vi "Main.vi"() -> ()   [LabVIEW 2016]
uses:
  Typedef/INS Data.ctl
  <vilib>/FPGAPlugInAG/roboRIO/niLvFpga_Open_roboRIO.vi
  <vilib>/rvi/interface/common/dynamic/niFpgaDynamicAddResources.vi
  <vilib>/FPGAPlugInAG/Dynamic/niLvFpga_Reset_Dynamic.vi
  <vilib>/Utility/error.llb/Error Cluster From Error Code.vi
  <vilib>/rvi/errors/niLvFpgaAdjustHostInterfaceError.vi
  <vilib>/myRIO/Common/Instrument Driver Framework/Utilities/vis/FPGA Ref Manager.vi
  <vilib>/myRIO/Common/Instrument Driver Framework/Utilities/vis/Ref Counter.vi
  <vilib>/FPGAPlugInAG/Dynamic/niLvFpga_Run_Dynamic.vi
  Shared resoruces/gear.vi
  Shared resoruces/Front Panel Control Variables.vi
  <vilib>/rvi/interface/nirviOpenFPGA/nirviOpenFPGA.xnode
  FPGA Bitfiles/AutoBikeMainFPGAbitfile.lvbitx
  <vilib>/rvi/interface/nirviMethod/nirviMethod.xnode
  <vilib>/rvi/interface/nirviReadWriteControl/nirviReadWriteControl.xnode
  <vilib>/rvi/interface/Simulation/niFpgaSimulationCallBeginRW.vi
  NiFpgaLv.dll
  <vilib>/myRIO/Instrument Drivers/Utilities/Utilities.lvlib
  Shared resoruces/Shared resources RT.lvlib
panel:
  in  "Reset Errors":bool
  in  "Send vel":bool
  in  "VEL":u16=850
  in  "UseGPS":bool=TRUE
  in  "Gear":enum16{"7", "6", "5", "4", "3", "2", "1"}(ring)=enum."3"
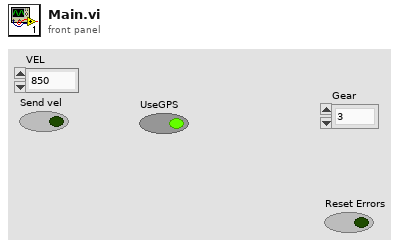
[diagram p1: front panel]
types:
  T1 = typedef "INS Data.ctl" = cluster{"Yaw":sgl, "Pitch":sgl, "Roll":sgl, "Lat":dbl, "Long":dbl, "Alt":dbl, "North":dbl, "East":dbl, "Down":dbl, "PosU":dbl, "VelU":dbl}
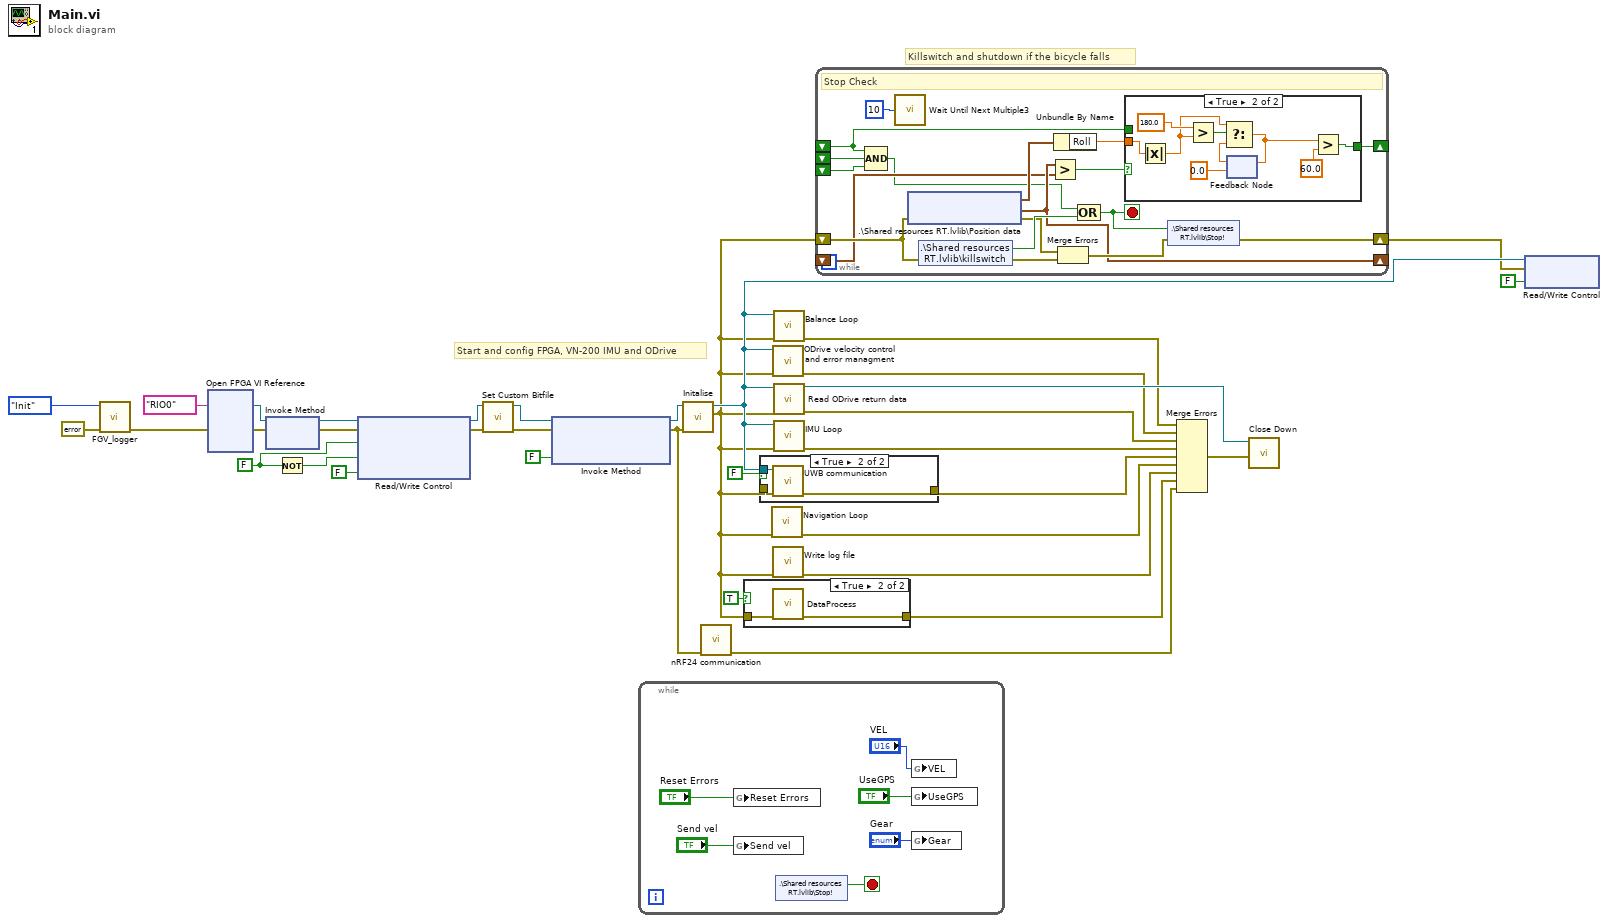
[diagram p0: block diagram]
diagram:
  w26 = FALSE ("Steering motor on?")
  # "Killswitch and shutdown if the bicycle falls"
  # "Start and config FPGA, VN-200 IMU and ODrive"
  n1 = call "FGV_logger.vi"("error in"=errorcluster {"status"=FALSE, "code"=0, "source"=""}, "Command"=enum16{"Update", "Log", "Init"}."Init") -> ("error out"=w32:errorcluster)  [unwired: 9 in]
  n2 = xnode "Open FPGA VI Reference"("error in"=w32, "resource name"=tag "RIO0") -> ("FPGA VI Reference Out"=w17:refnum<k20>, "error out"=w18:errorcluster)
  n3 = xnode "Invoke Method"("FPGA VI Reference In"=w17, "error in"=w18) -> ("FPGA VI Reference Out"=w30:refnum<k20>, "error out"=w29:errorcluster)
  n4 = Not(x=w26) -> (.not. x?=w27:bool)
  n5 = xnode "Read/Write Control"("FPGA VI Reference In"=w30, "error in"=w29, "Comm LED Green"=w26, "Comm LED Red"=w27, "MotorsON"=FALSE ("Rear wheel motor OFF?")) -> ("FPGA VI Reference Out"=w23:refnum<k20>, "error out"=w24:errorcluster)
  n6 = call <vilib>:"Set Custom Bitfile.vi"("error in (no error)"=w24, "Custom FPGA Reference In"=w23) -> ("error out"=w22:errorcluster, "Custom FPGA Reference Out"=w21:refnum<k20>)  [unwired: 8 in]
  n7 = xnode "Invoke Method"("FPGA VI Reference In"=w21, "error in"=w22, "Wait Until Done (F)"=FALSE) -> ("FPGA VI Reference Out"=w19:refnum<k20>, "error out"=w20:errorcluster)
  n8 = while {
    stop <- w36 stop-if-true
    n9 = global write "Front Panel Control Variables.vi" "Reset Errors"("Reset Errors") -> ()
    n10 = global write "Front Panel Control Variables.vi" "Send vel"("Send vel") -> ()
    n11 = shared-variable ".\\Shared resources RT.lvlib\\Stop!"() -> (w36:bool)  [unwired: 1 in, 1 out]
    n12 = global write "Front Panel Control Variables.vi" "VEL"("VEL") -> ()
    n13 = global write "Front Panel Control Variables.vi" "UseGPS"("UseGPS") -> ()
    n14 = global write "gear.vi" "Gear"("Gear") -> ()
  }
  n15 = call "Initalise.vi"("error in (no error)"=w20, "FPGA Interface"=w19) -> ("Error out"=w5:errorcluster, "FPGA VI Reference Out"=w7:refnum<k20>)  [unwired: 7 in, 1 out]
  n16 = call "nRF24 communication.vi"("error in (no error)"=w20) -> ("error out"=w4:errorcluster)  [unwired: 10 in]
  n17 = case shown="True" TRUE {
    tunnel: w5 -> [w42 w44]
    tunnel: [w42 w43] -> w3
    frame False {
    }
    frame True {
      n18 = call "DataProcess.vi"("error in (no error)"=w44) -> ("error out"=w43:errorcluster)  [unwired: 10 in]
    }
  }
  n19 = case shown="True" FALSE {
    tunnel: [w45 w48] -> w11
    tunnel: w7 -> [_ w47]
    tunnel: w5 -> [w45 w46]
    frame False {
    }
    frame True {
      n20 = call "UWB communication.vi"("error in (no error)"=w46, "FPGA VI Reference In"=w47) -> ("error out"=w48:errorcluster)  [unwired: 8 in, 1 out]
    }
  }
  n21 = call "Navigation Loop.vi"("error in (no error)"=w5) -> ("error out"=w10:errorcluster)  [unwired: 10 in]
  n22 = call "ODrive velocity control and error managment.vi"("error in (no error)"=w5, "Refnum in"=w7) -> ("Error out"=w14:errorcluster)  [unwired: 8 in, 1 out]
  n23 = call "Write log file.vi"("error in (no error)"=w5) -> ("error out"=w9:errorcluster)  [unwired: 10 in]
  n24 = call "Balance Loop.vi"("error in (no error)"=w5, "Refnum in"=w7) -> ("error out"=w15:errorcluster)  [unwired: 8 in, 1 out]
  n25 = call "Read ODrive return data.vi"("error in (no error)"=w5, "Refnum in"=w7) -> ("error out"=w13:errorcluster, "Refnum out"=w16:refnum<k20>)  [unwired: 8 in]
  n26 = call "IMU Loop.vi"("error in (no error)"=w5, "FPGA ref in"=w7) -> ("error out"=w12:errorcluster)  [unwired: 9 in]
  n27 = while {
    shift-right: [w66] -> w6
    shift-left: w5 -> [w62]
    shift-right: [w57] -> _
    shift-left: _ -> [w56]
    shift-right: [w53] -> _
    shift-left: _ -> [w51]
    shift-left: _ -> [w52]
    shift-left: _ -> [w50]
    stop <- w59 stop-if-true
    # "Stop Check"
    n28 = Compound Arithmetic op=AND(w51, w52, w50) -> (w49:bool)
    n29 = call "Wait Until Next Multiple3"("Count(mSec)"=u32 10) -> ()  [unwired: 1 out]
    n30 = shared-variable ".\\Shared resources RT.lvlib\\Position data"(error in=w62) -> (w60:T1, error out=w61:errorcluster, w57:timestamp)
    n31 = shared-variable ".\\Shared resources RT.lvlib\\killswitch"(error in=w62) -> (w65:bool, error out=w63:errorcluster)
    n32 = Greater?(x=w57, y=w56) -> (0:w55:bool)
    n33 = Unbundle By Name(w60) -> ("Roll"=w54:sgl)
    n34 = Merge Errors(w61, w63) -> (w64:errorcluster)
    n35 = Compound Arithmetic op=OR(w49, w65) -> (w59:bool)
    n36 = case shown="True" w55 {
      tunnel: w54 -> [_ w70]
      tunnel: [w67 w75] -> w53
      tunnel: w51 -> [w67 _]
      frame False {
      }
      frame True {
        n37 = Absolute Value(x=w70) -> (abs(x)=w69:sgl)
        n38 = Greater?(x=sgl 180.0 ("upper limit"), y=w69) -> (0:w74:bool)
        n39 = feedback #1(sgl 0.0 ("Roll")) -> (w72:sgl)
        n40 = Select(t=w69, s=w74, f=w72) -> (s? t:f=w68:sgl)
        n41 = feedback-in #1(w68) -> ()
        n42 = Greater?(x=w68, y=sgl 60.0) -> (0:w75:bool)
      }
    }
    n43 = shared-variable ".\\Shared resources RT.lvlib\\Stop!"(w59, error in=w64) -> (error out=w66:errorcluster)
  }
  n44 = Merge Errors(w15, w14, w13, w12, w11, w10, w9, w3, w4) -> (w34:errorcluster)
  n45 = call "Close Down.vi"("error in (no error)"=w34, "FPGA Interface"=w16) -> ()  [unwired: 9 in, 1 out]
  n46 = xnode "Read/Write Control"("FPGA VI Reference In"=w7, "error in"=w6, "MotorsON"=FALSE) -> ()  [unwired: 2 out]
